vi "LVClass_Camera start acquisition.vi"(0 "Camera in":refnum<class "Camera.lvclass">, 5 "synchronisation_mode":enum16{"synchronous", "asynchronous"}(ring), 7 "acquisition_mode":enum16{"last_image", "new_image"}(ring), 11 "error in (no error)":errorcluster) -> (4 "Camera out":refnum<class "Camera.lvclass">, 15 "error out":errorcluster)   [LabVIEW 2020, in "Camera.lvclass"]
doc: "Start acquisition.\n\n<B>CameraIn</B> : Camera object.\n<B>CameraOut</B> : Camera object.\n<B>acquisition_mode</B> : Acquisition mode : can be 0 (last_image) or 1 (new_image).\n<B>synchronization_mode</B> : Synchronisation mode : can be 0 (synchronous) or 1 (asynchronous)."
uses:
  Camera.lvclass
  Controls/CameraAcquisitionState.ctl
  Camera.lvclass/Camera.ctl
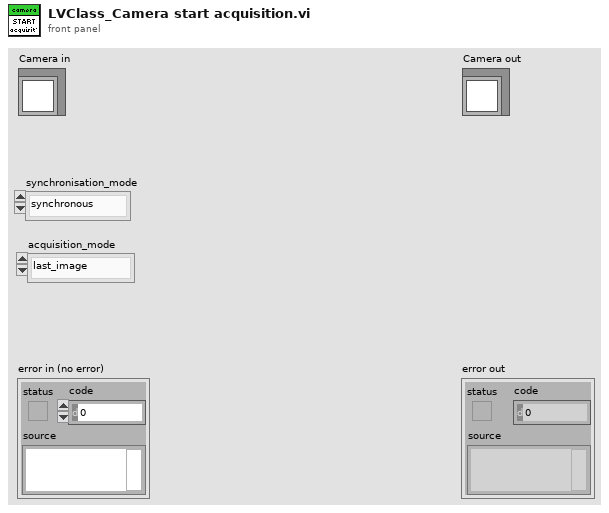
[diagram p1: front panel]
types:
  T1 = typedef "CameraAcquisitionState.ctl" = enum16{"Stop", "Live"}
  T2 = typedef "ClassID.ctl" = i64
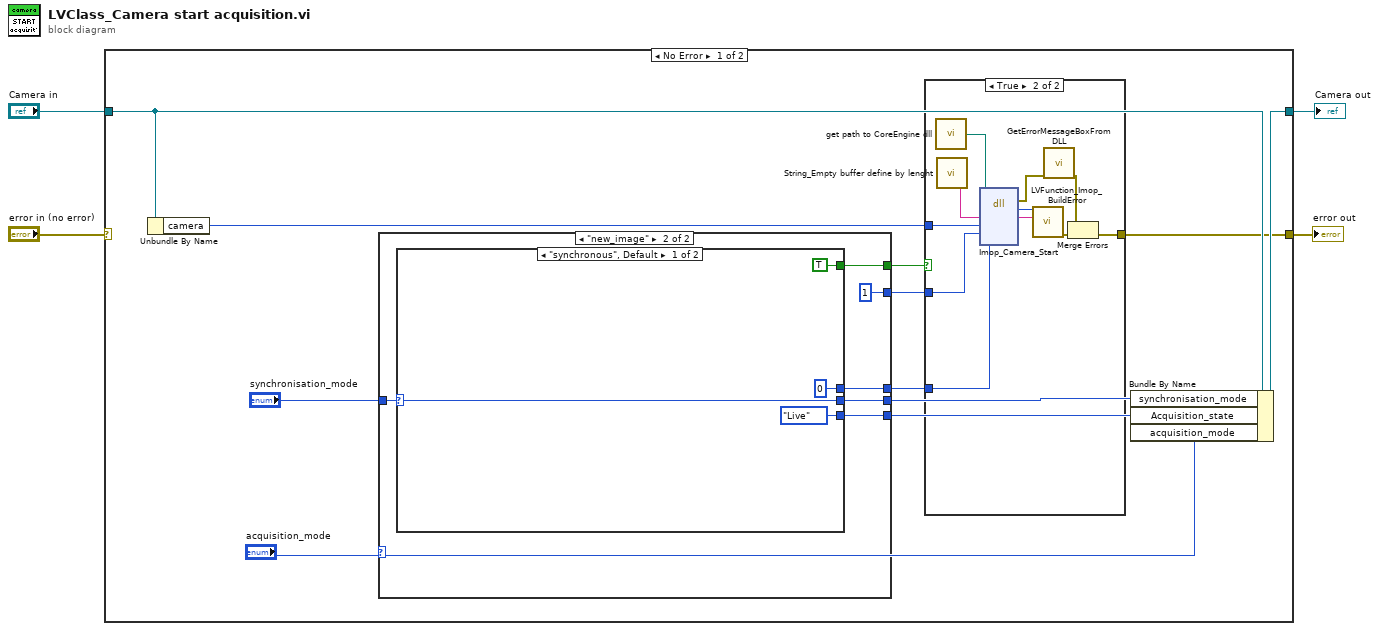
[diagram p0: block diagram]
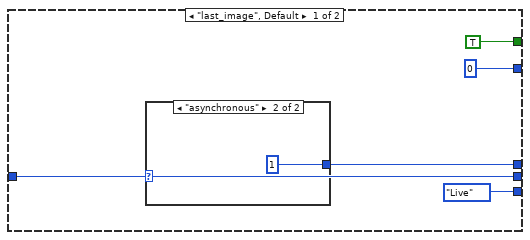
[diagram p2: hidden frame]
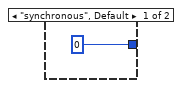
[diagram p3: hidden frame]
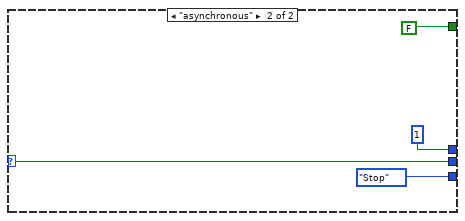
[diagram p4: hidden frame]
diagram:
  n1 = case shown="No Error" "error in (no error)" {
    selector: "error in (no error)" -> [_ w50]
    tunnel: [w11 w50] -> w3
    tunnel: [w12 w49] -> w1
    tunnel: "Camera in" -> [w13 w49]
    frame No Error {
      n2 = Unbundle By Name(w13) -> ("camera"=w15:T2)
      n3 = case shown="\"new_image\"" "acquisition_mode" {
        tunnel: [0 1] -> w14
        tunnel: "synchronisation_mode" -> [w18 w26]
        tunnel: [w19 w25] -> w10
        tunnel: [w18 w27] -> w9
        tunnel: [CameraAcquisitionState."Live" ("Acquisition_state") w24] -> w7
        tunnel: [TRUE w23] -> w6
        frame "last_image", Default {
          n4 = case shown="\"asynchronous\"" w18 {
            tunnel: [0 1] -> w19
            frame "synchronous", Default {
            }
            frame "asynchronous" {
            }
          }
        }
        frame "new_image" {
          n5 = case shown="\"synchronous\", Default" w26 {
            selector: w26 -> [w32 w36]
            tunnel: [w32 w36] -> w27
            tunnel: [0 1] -> w25
            tunnel: [CameraAcquisitionState."Live" ("Acquisition_state") CameraAcquisitionState."Stop" ("Acquisition_state")] -> w24
            tunnel: [TRUE FALSE] -> w23
            frame "synchronous", Default {
            }
            frame "asynchronous" {
            }
          }
        }
      }
      n6 = case shown="True" w6 {
        tunnel: w15 -> [_ w48]
        tunnel: w14 -> [_ w44]
        tunnel: [errorcluster {"status"=FALSE, "code"=0, "source"=""} ("error IO") w41] -> w11
        tunnel: w10 -> [_ w40]
        frame False {
        }
        frame True {
          n7 = call "get path to CoreEngine dll.vi"() -> ("path to wavekit library"=w39:path)  [unwired: 14 in, 1 out]
          n8 = call "String_Empty buffer define by lenght.vi"() -> ("Empty buffer"=w38:string)  [unwired: 1 in]
          n9 = dll-call lib="D:/2_trunk/Soft_haso/ImOpCoreEngine4_LV2011/DLLs/ImopEngine4_vc100.dll" fn="Imop_Camera_Start"(path in=w39, "message"=w38, "objet"=w48, "acquisition_mode"=w44, "synchronization_mode"=w40) -> (error out=w45:errorcluster, "return type"=w46:i32, "message"=w47:string)  [unwired: 5 in, 1 out]
          n10 = call "LVFunction_Imop_BuildError.vi"("code"=w46, "String to Prepend to source (\"\")"=w47) -> ("error out"=w42:errorcluster)  [unwired: 13 in]
          n11 = call "GetErrorMessageBoxFromDLL.vi"("error IN"=w45) -> ("error OUT"=w43:errorcluster)  [unwired: 10 in]
          n12 = Merge Errors(w43, w42) -> (w41:errorcluster)
        }
      }
      n13 = Bundle By Name(cluster=w13, "synchronisation_mode"=w9, "Acquisition_state"=w7, "acquisition_mode"="acquisition_mode") -> (w12:refnum<class "Camera.lvclass">)
    }
    frame Error {
    }
  }
  "error out" <- w3
  "Camera out" <- w1
